vi "Upload Next.vi"(8 "error in (no error)":errorcluster, 10 "Step Num":u16, 11 "SLM_Controller in":refnum<class "SLM_Controller.lvclass">) -> (0 "error out":errorcluster, 3 "SLM_Controller out":refnum<class "SLM_Controller.lvclass">)   [LabVIEW 2023, in "SLM_Controller.lvlib" / "SLM_Controller.lvclass"]
uses:
  SLM_Controller.lvclass
  SLM_Controller.lvclass/SLM_Controller.ctl
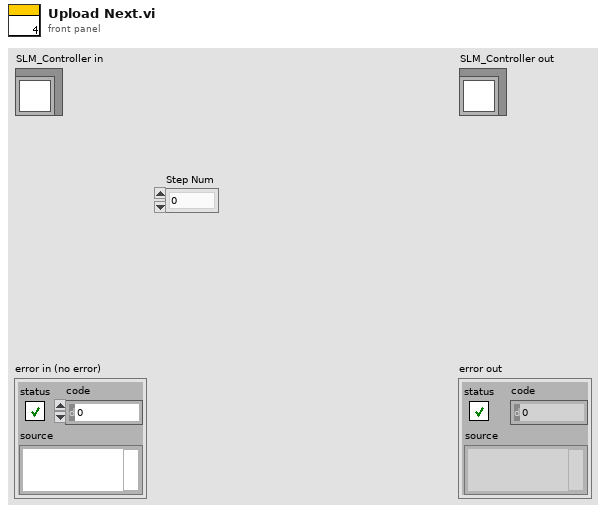
[diagram p1: front panel]
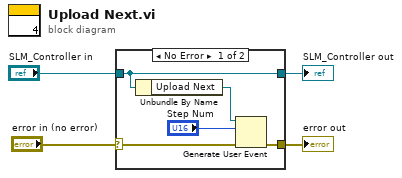
[diagram p0: block diagram]
diagram:
  n1 = case shown="No Error" "error in (no error)" {
    selector: "error in (no error)" -> [w7 w11]
    tunnel: [w6 w11] -> w3
    tunnel: [w9 w10] -> w1
    tunnel: "SLM_Controller in" -> [w9 w10]
    frame No Error {
      n2 = Unbundle By Name(w9) -> ("Upload Next"=w8:refnum<user-event>)
      n3 = Generate User Event(user event=w8, event data cluster="Step Num", error in=w7) -> (error out=w6:errorcluster)  [unwired: 1 in, 1 out]
    }
    frame Error {
    }
  }
  "error out" <- w3
  "SLM_Controller out" <- w1
